vi "CheckSchemaVerions.vi"(8 "error in (no error)":errorcluster, 10 "ValidSchemaVersions":string[](array[string])=["00.00.01"], 11 "schemaVersion":string) -> (0 "error out":errorcluster)   [LabVIEW 2026, in "Lumberjack.lvlib"]
uses:
  Lumberjack.lvlib
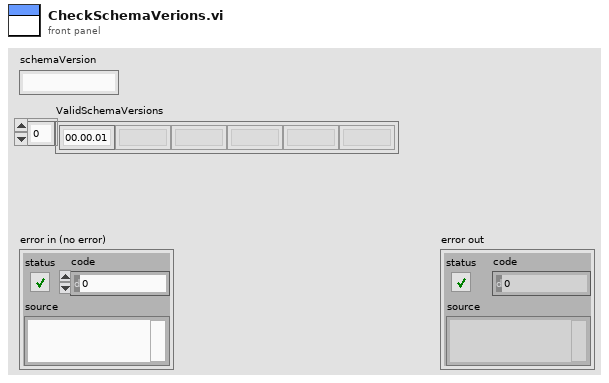
[diagram p1: front panel]
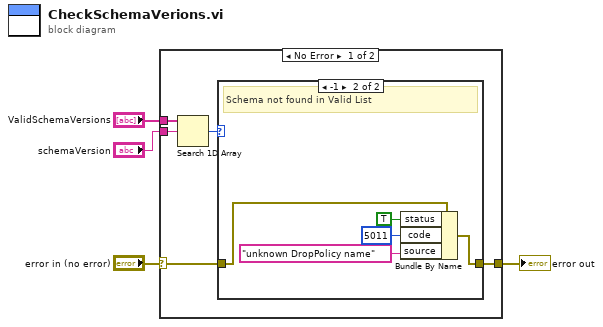
[diagram p0: block diagram]
diagram:
  n1 = case shown="No Error" "error in (no error)" {
    selector: "error in (no error)" -> [w6 w16]
    tunnel: [w9 w16] -> w4
    tunnel: "schemaVersion" -> [w8 _]
    tunnel: "ValidSchemaVersions" -> [w5 _]
    frame No Error {
      n2 = Search 1D Array(1D array=w5, element=w8) -> (index of element=w7:i32)  [unwired: 1 in]
      n3 = case shown="-1" w7 {
        tunnel: w6 -> [w10 w15]
        tunnel: [w10 w14] -> w9
        frame Default {
          # "Schema found in Valid List"
        }
        frame -1 {
          # "Schema not found in Valid List"
          n4 = Bundle By Name(cluster=w15, "status"=TRUE, "code"=5011, "source"="unknown DropPolicy name") -> (w14:errorcluster)
        }
      }
    }
    frame Error {
    }
  }
  "error out" <- w4
